vi "Decode CSV to 2D Array.vi"(6 "Delimiter (,)":string=",", 8 "error in":errorcluster, 11 "Spreadsheet String":string) -> (0 "error out":errorcluster, 3 "2D Array":string[][](array[string]))   [LabVIEW 2024, in "dataLogger.lvlib"]
doc: "This converts a Spreadsheet String to a 2D String array even when an individual cell contains characters which are not supported by the built-in Spreadsheet String to Array function (like new line characters)."
uses:
  dataLogger.lvlib
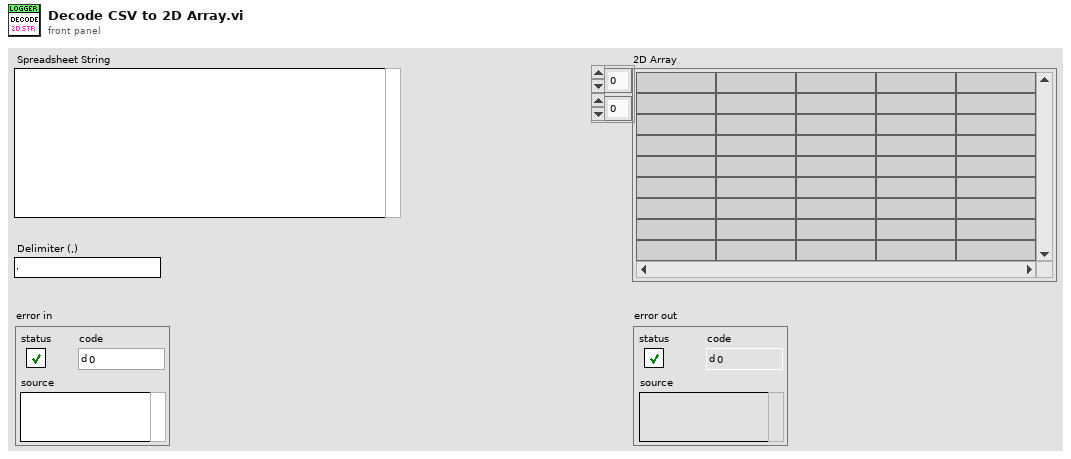
[diagram p1: front panel]
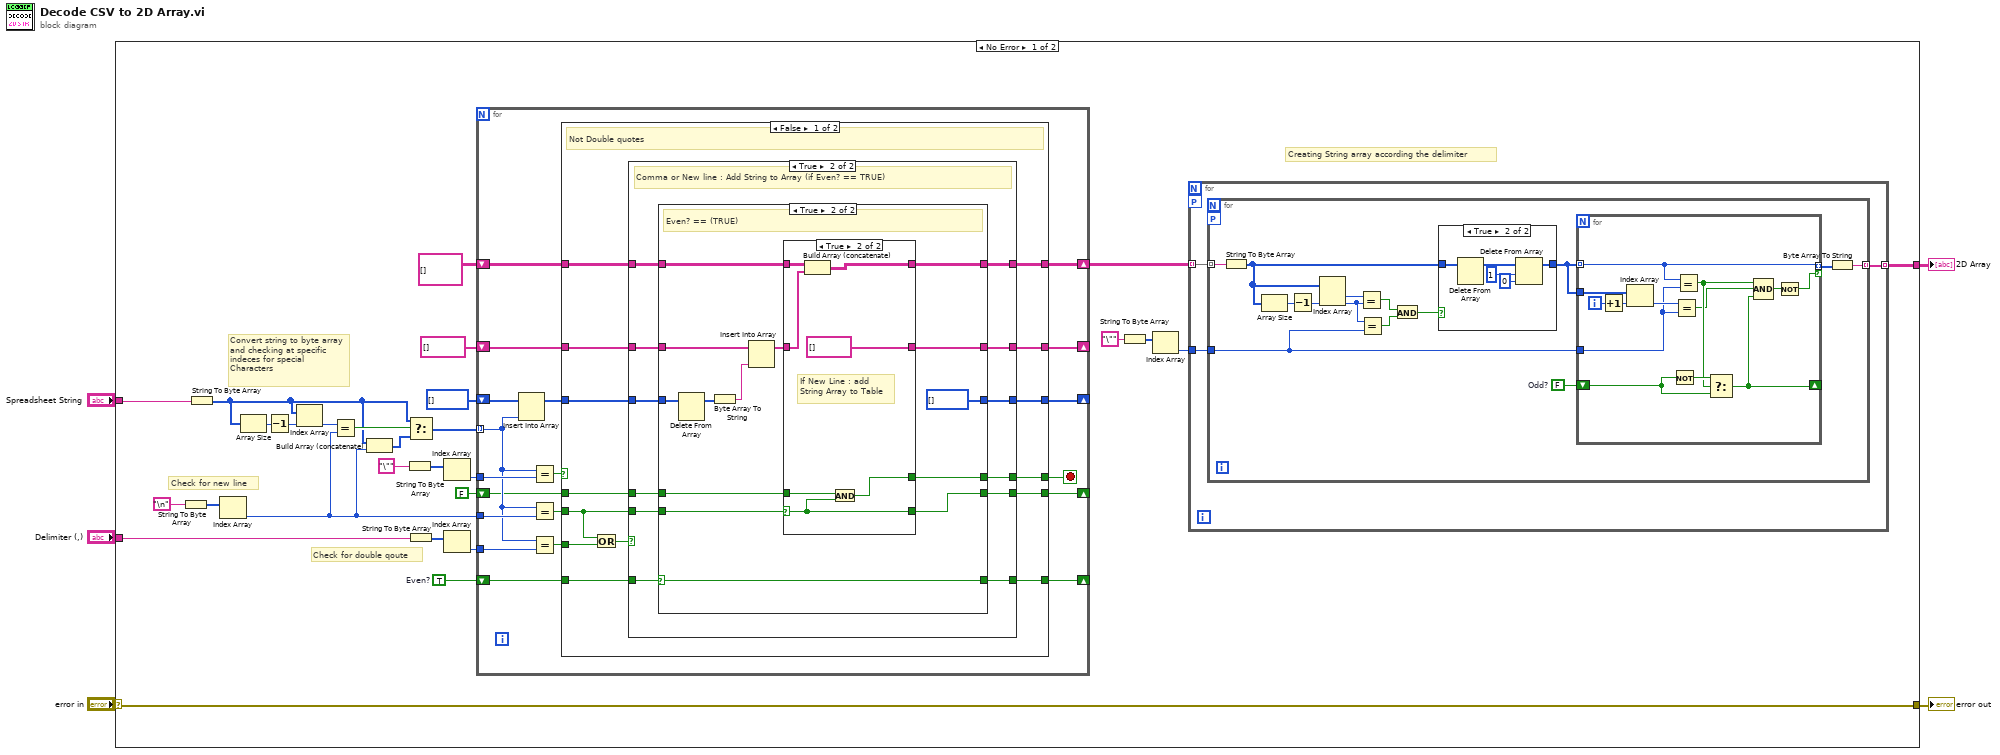
[diagram p0: block diagram]
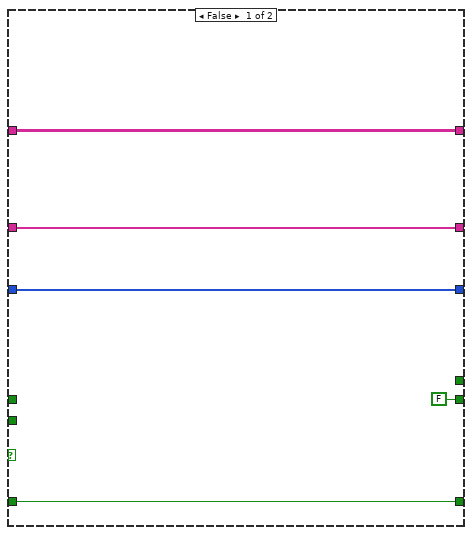
[diagram p3: hidden frame]
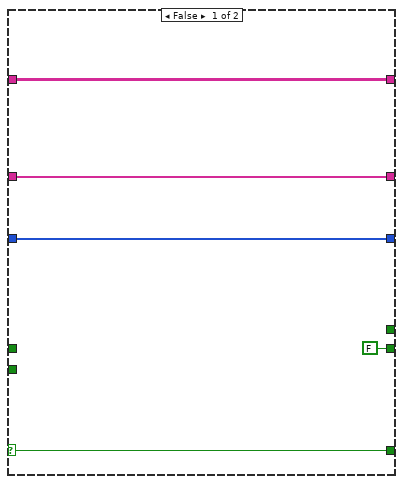
[diagram p4: hidden frame]
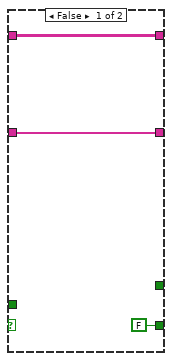
[diagram p5: hidden frame]
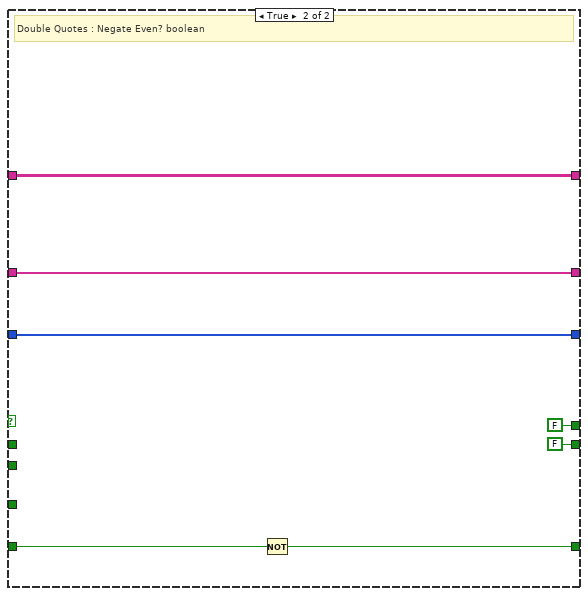
[diagram p6: hidden frame]
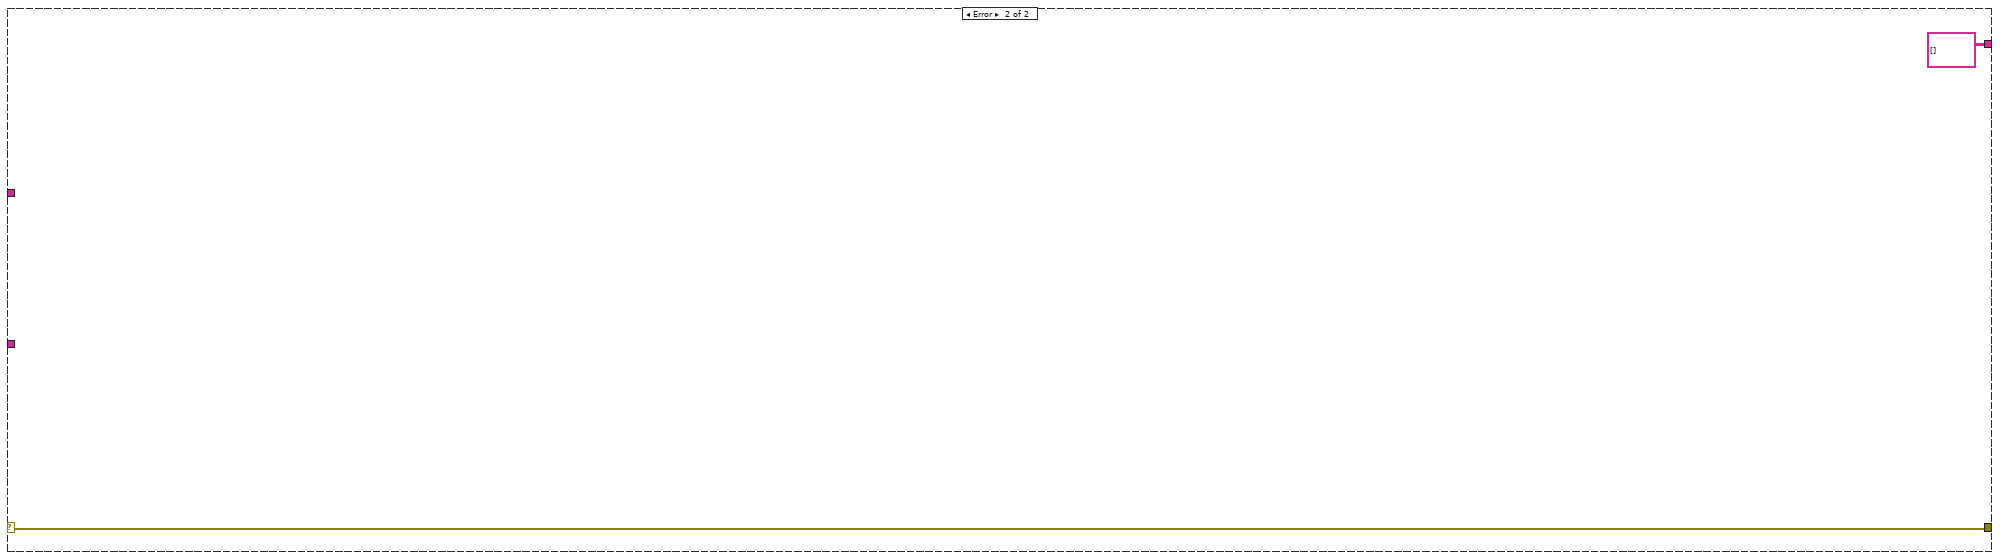
[diagram p7: hidden frame]
diagram:
  n1 = case shown="No Error" "error in" {
    selector: "error in" -> [w7 w157]
    tunnel: "Delimiter (,)" -> [w31 _]
    tunnel: [w20 string[][] []] -> w4
    tunnel: "Spreadsheet String" -> [w16 _]
    tunnel: [w7 w157] -> w1
    frame No Error {
      w25 = TRUE  # Even?
      # "Creating String array according the delimiter"
      # "Convert string to byte array and checking at specific indeces for special Characters"
      # "Check for new line"
      # "Check for double qoute"
      n2 = String To Byte Array(string="\n") -> (unsigned byte array=w29:u8[])
      n3 = String To Byte Array(string=w16) -> (unsigned byte array=w9:u8[])
      n4 = Index Array(array=w29) -> (element=w8:u8)  [unwired: 1 in]
      n5 = Array Size(array=w9) -> (size(s)=w15:i32)
      n6 = Decrement(x=w15) -> (x-1=w14:i32)
      n7 = Index Array(array=w9, index=w14) -> (element=w13:u8)
      n8 = Equal?(x=w13, y=w8) -> (x = y?=w12:bool)
      n9 = Build Array (concatenate)(w9, w8) -> (w10:u8[])
      n10 = String To Byte Array(string="\"") -> (unsigned byte array=w30:u8[])
      n11 = String To Byte Array(string=w31) -> (unsigned byte array=w28:u8[])
      n12 = Select(t=w9, s=w12, f=w10) -> (s? t:f=w11:u8[])
      n13 = Index Array(array=w30) -> (element=w27:u8)  [unwired: 1 in]
      n14 = Index Array(array=w28) -> (element=w26:u8)  [unwired: 1 in]
      n15 = for {
        tunnel: w11 -> [w73] mode=indexing
        tunnel: w27 -> [w76]
        tunnel: w8 -> [w75]
        tunnel: w26 -> [w74]
        shift-right: [w84] -> _
        shift-left: w25 -> [w85]
        shift-right: [w82] -> _
        shift-left: u8[] [] -> [w81]
        shift-right: [w79] -> _
        shift-left: string[] [] -> [w80]
        shift-right: [w77] -> w33
        shift-left: string[][] [] -> [w78]
        shift-right: [w72] -> _
        shift-left: FALSE -> [w71]
        stop <- w70 stop-if-true
        n16 = Insert Into Array(array=w81, new element=w73) -> (w83:u8[])  [unwired: 1 in]
        n17 = Equal?(x=w73, y=w76) -> (x = y?=w88:bool)
        n18 = Equal?(x=w73, y=w75) -> (x = y?=w87:bool)
        n19 = Equal?(x=w73, y=w74) -> (x = y?=w86:bool)
        n20 = case shown="False" w88 {
          tunnel: w87 -> [w92 _]
          tunnel: w86 -> [w93 _]
          tunnel: w85 -> [w102 w155]
          tunnel: [w101 w154] -> w84
          tunnel: w83 -> [w100 w151]
          tunnel: [w99 w151] -> w82
          tunnel: w80 -> [w98 w153]
          tunnel: [w97 w153] -> w79
          tunnel: w78 -> [w96 w152]
          tunnel: [w95 w152] -> w77
          tunnel: [w91 FALSE] -> w72
          tunnel: w71 -> [w90 _]
          tunnel: [w89 FALSE] -> w70
          frame False {
            # "Not Double quotes"
            n21 = Or(x=w92, y=w93) -> (x .or. y?=w94:bool)
            n22 = case shown="True" w94 {
              tunnel: w102 -> [w106 w119]
              tunnel: [w106 w114] -> w101
              tunnel: w100 -> [w105 w116]
              tunnel: [w105 w115] -> w99
              tunnel: w98 -> [w104 w118]
              tunnel: [w104 w117] -> w97
              tunnel: w96 -> [w107 w113]
              tunnel: [w107 w112] -> w95
              tunnel: w92 -> [_ w111]
              tunnel: [FALSE w110] -> w91
              tunnel: w90 -> [_ w109]
              tunnel: [_ w108] -> w89
              frame False {
              }
              frame True {
                # "Comma or New line : Add String to Array (if Even? == TRUE)"
                n23 = case shown="True" w119 {
                  selector: w119 -> [w122 w138]
                  tunnel: [w124 w135] -> w117
                  tunnel: w118 -> [w124 w133]
                  tunnel: [w123 u8[] []] -> w115
                  tunnel: w116 -> [w123 w129]
                  tunnel: [w122 w138] -> w114
                  tunnel: w113 -> [w121 w137]
                  tunnel: [w121 w134] -> w112
                  tunnel: w111 -> [_ w128]
                  tunnel: [FALSE w127] -> w110
                  tunnel: w109 -> [_ w126]
                  tunnel: [_ w125] -> w108
                  frame False {
                  }
                  frame True {
                    # "Even? == (TRUE)"
                    n24 = Delete From Array(array=w129) -> (array with subset deleted=w130:u8[])  [unwired: 2 in, 1 out]
                    n25 = Byte Array To String(unsigned byte array=w130) -> (string=w131:string)
                    n26 = Insert Into Array(array=w133, new element=w131) -> (w132:string[])  [unwired: 1 in]
                    n27 = case shown="True" w128 {
                      selector: w128 -> [_ w143]
                      tunnel: w137 -> [w141 w148]
                      tunnel: [w140 string[] []] -> w135
                      tunnel: [w141 w146] -> w134
                      tunnel: w132 -> [w140 w145]
                      tunnel: [FALSE w143] -> w127
                      tunnel: w126 -> [_ w144]
                      tunnel: [_ w142] -> w125
                      frame False {
                      }
                      frame True {
                        # "If New Line : add String Array to Table"
                        n28 = Build Array (concatenate)(w148, w145) -> (w146:string[][])
                        n29 = And(x=w144, y=w143) -> (x .and. y?=w142:bool)
                      }
                    }
                  }
                }
              }
            }
          }
          frame True {
            # "Double Quotes : Negate Even? boolean"
            n30 = Not(x=w155) -> (.not. x?=w154:bool)
          }
        }
      }
      n31 = String To Byte Array(string="\"") -> (unsigned byte array=w18:u8[])
      n32 = Index Array(array=w18) -> (element=w17:u8)  [unwired: 1 in]
      n33 = for {
        tunnel: w33 -> [w36] mode=indexing
        tunnel: w17 -> [w35]
        tunnel: [w34] -> w20 mode=indexing
        workers-P: _ -> [_]
        n34 = for {
          tunnel: w36 -> [w50] mode=indexing
          tunnel: w35 -> [w40]
          tunnel: [w38] -> w34 mode=indexing
          workers-P: _ -> [_]
          w37 = FALSE  # Odd?
          n35 = String To Byte Array(string=w50) -> (unsigned byte array=w42:u8[])
          n36 = Array Size(array=w42) -> (size(s)=w49:i32)
          n37 = Decrement(x=w49) -> (x-1=w48:i32)
          n38 = Index Array(array=w42, index #2=w48) -> (element #1=w47:u8, element #2=w46:u8)  [unwired: 1 in]
          n39 = Equal?(x=w47, y=w46) -> (x = y?=w44:bool)
          n40 = Equal?(x=w46, y=w40) -> (x = y?=w45:bool)
          n41 = And(x=w44, y=w45) -> (x .and. y?=w43:bool)
          n42 = case shown="True" w43 {
            tunnel: w42 -> [w64 w69]
            tunnel: [w64 w67] -> w41
            frame False {
            }
            frame True {
              n43 = Delete From Array(array=w69) -> (array with subset deleted=w68:u8[])  [unwired: 2 in, 1 out]
              n44 = Delete From Array(array=w68, length=1, index=0) -> (array with subset deleted=w67:u8[])  [unwired: 1 out]
            }
          }
          n45 = for {
            tunnel: w41 -> [w58] mode=indexing
            tunnel: w41 -> [w63]
            tunnel: w40 -> [w59]
            tunnel: [w58] -> w39 mode=indexing if=w57
            shift-right: [w52] -> _
            shift-left: w37 -> [w56]
            i -> [w62]
            n46 = Increment(x=w62) -> (x+1=w61:i32)
            n47 = Index Array(array=w63, index=w61) -> (element=w60:u8)
            n48 = Not(x=w56) -> (.not. x?=w55:bool)
            n49 = Equal?(x=w60, y=w59) -> (x = y?=w53:bool)
            n50 = Equal?(x=w58, y=w59) -> (x = y?=w54:bool)
            n51 = Select(t=w55, s=w54, f=w56) -> (s? t:f=w52:bool)
            n52 = Compound Arithmetic op=AND(w54, w53, w52) -> (w51:bool)
            n53 = Not(x=w51) -> (.not. x?=w57:bool)
          }
          n54 = Byte Array To String(unsigned byte array=w39) -> (string=w38:string)
        }
      }
    }
    frame Error {
    }
  }
  "2D Array" <- w4
  "error out" <- w1
